vi "find first peak - percentage (SubVI).vi"(8 "width":i32=3, 9 "1st peak ratio\n(%max)":dbl=0.1, 10 "Array":dbl[](array[numeric])) -> (0 "amplitude":dbl, 1 "actual ratio":dbl, 2 "#peaks":i32, 3 "Index":dbl)   [LabVIEW 2012]
uses:
  <vilib>/Analysis/NI_AAL_SigProc.lvlib
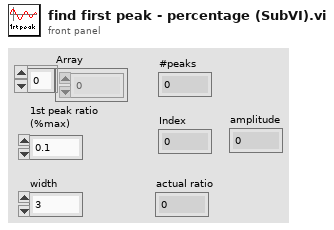
[diagram p1: front panel]
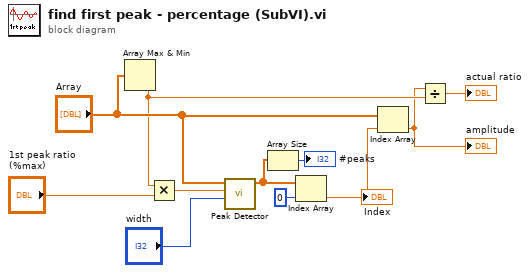
[diagram p0: block diagram]
diagram:
  n1 = Array Max & Min(array="Array") -> (max value=w3:dbl)  [unwired: 3 out]
  n2 = Multiply(x=w3, y="1st peak ratio\n(%max)") -> (x*y=w6:dbl)
  n3 = call <vilib>:"Peak Detector.vi"("width"="width", "threshold"=w6, "X"="Array") -> ("Locations"=w8:dbl[])  [unwired: 4 in, 4 out]
  n4 = Array Size(array=w8) -> (size(s)=→"#peaks":i32)
  n5 = Index Array(array=w8, index=0) -> (element=w5:dbl)
  "Index" <- w5
  n6 = Index Array(array="Array", index=w5) -> (element=w2:dbl)
  "amplitude" <- w2
  n7 = Divide(x=w2, y=w3) -> (x/y=→"actual ratio":dbl)
